vi "Draw.vi"(8 "error in (no error)":errorcluster, 11 "Gradient Rectangle in":refnum<class "Gradient Rectangle.lvclass">) -> (0 "error out":errorcluster, 2 "Picture":picture, 3 "Gradient Rectangle out":refnum<class "Gradient Rectangle.lvclass">)   [LabVIEW 2016, in "Gradient Rectangle.lvclass"]
uses:
  Gradient Rectangle.lvclass
  C:/Program Files (x86)/National Instruments/LabVIEW 2016/vi.lib/LIEF/Forms/Shape/Shape.lvclass
  Gradient Rectangle.lvclass/Gradient Rectangle.ctl
  <vilib>/LIEF/Forms/Shape/Shape.lvclass/Shape.ctl
  <vilib>/LIEF/Forms/Shape/Read Color.vi
  <vilib>/LIEF/Forms/Layered Shape/Layered Shape.lvclass
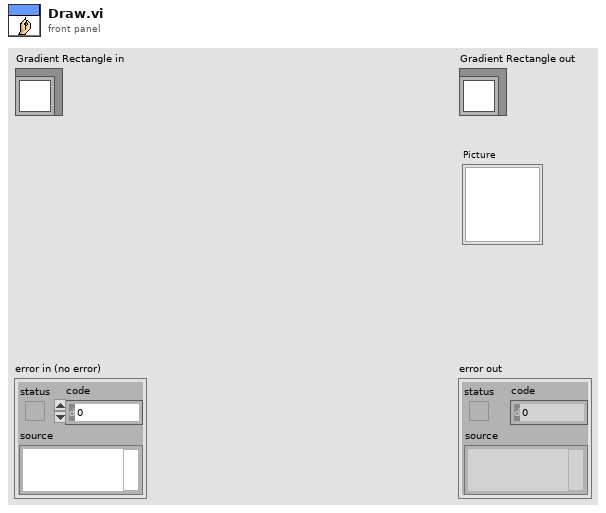
[diagram p1: front panel]
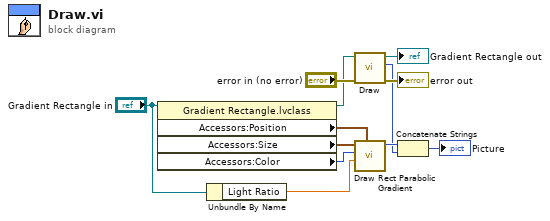
[diagram p0: block diagram]
diagram:
  n1 = property class="Gradient Rectangle.lvclass"(reference="Gradient Rectangle in") -> (reference out=w5:refnum<class "Gradient Rectangle.lvclass">, "Accessors:Position"=w1:cluster{"Left":i32, "Top":i32}, "Accessors:Size"=w2:cluster{"Width":i32, "Height":i32}, "Accessors:Color"=w3:u32)  [unwired: 1 in, 1 out]
  n2 = Unbundle By Name("Gradient Rectangle in") -> ("Light Ratio"=w9:dbl)
  n3 = call-parent "Draw.vi"("error in (no error)"="error in (no error)", "Layered Shape in"=w5) -> ("error out"=→"error out":errorcluster, "Picture"=w7:picture, "Layered Shape out"=→"Gradient Rectangle out":refnum<class "Gradient Rectangle.lvclass">)  [unwired: 7 in]
  n4 = call "Draw Rect Parabolic Gradient.vi"("Position"=w1, "Percentage(30)"=w9, "Color"=w3, "Size"=w2) -> ("2D Picture"=w8:picture)  [unwired: 7 in]
  n5 = Concatenate Strings(w8, w7) -> (→"Picture":picture)
